vi "SPI Slave Read Write Bytes.vi"(4 "TimeOutMs":i32, 5 "WriteDataLen":i32, 6 "pWriteData":u8[](array[numeric])=array[4097 elements], 7 "ReadDataLen":i32, 9 "pReadData":u8[](array[numeric])=array[4097 elements], 10 "SPIIndex":i32, 11 "DevHandle":i32) -> (1 "pReadData out":u8[](array[numeric]), 2 "function return":i32, 3 "pWriteData out":u8[](array[numeric]))   [LabVIEW 2010, in "usb2spi.lvlib"]
doc: "int WINAPI SPI_SlaveReadWriteBytes(int DevHandle,int SPIIndex,unsigned char *pReadData,int ReadDataLen,unsigned char *pWriteData,int WriteDataLen,int TimeOutMs);"
uses:
  usb2spi.lvlib
  USB2XXX/trunk/USB2XXX/USB2XXX/vs2010/Release/USB2XXX.dll
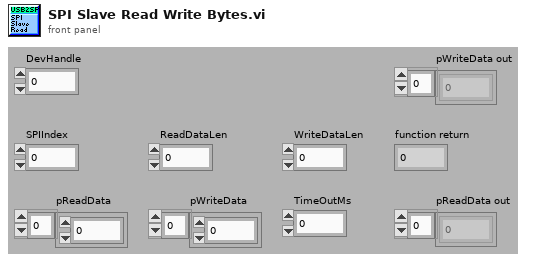
[diagram p1: front panel]
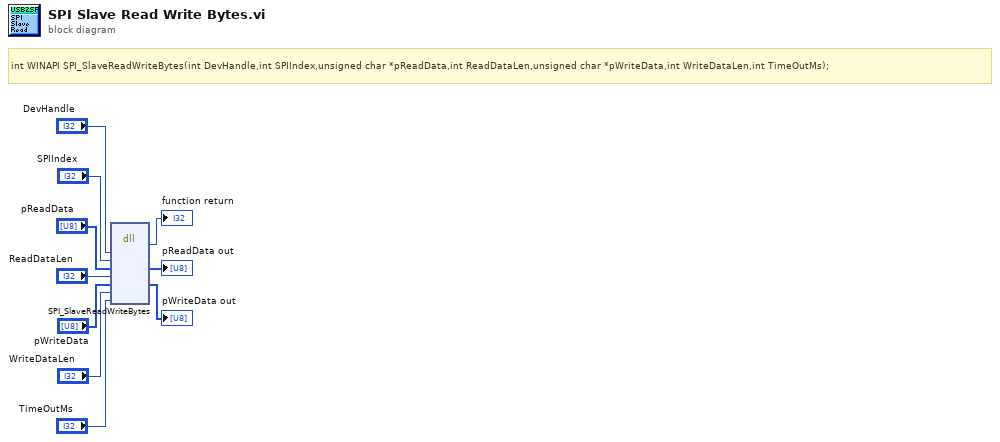
[diagram p0: block diagram]
diagram:
  # "int WINAPI SPI_SlaveReadWriteBytes(int DevHandle,int SPIIndex,unsigned char *pReadData,int ReadDataLen,unsigned char *pWriteData,int WriteDataLen,int TimeOutMs);"
  n1 = dll-call lib="E:/OtherWork/STM32/USB2XXX/trunk/USB2XXX/USB2XXX/vs2010/Release/USB2XXX.*" fn="SPI_SlaveReadWriteBytes"("DevHandle"="DevHandle", "SPIIndex"="SPIIndex", "pReadData"="pReadData", "ReadDataLen"="ReadDataLen", "pWriteData"="pWriteData", "WriteDataLen"="WriteDataLen", "TimeOutMs"="TimeOutMs") -> (→"function return":i32, "pReadData"=→"pReadData out":u8[], "pWriteData"=→"pWriteData out":u8[])  [unwired: 8 in, 2 out]
